vi "PQcopyOut.vi"(8 "error in (no error)":errorcluster, 9 "count":u32, 10 "query":string, 11 "conn":u32) -> (0 "database_status_message":T1, 1 "data":string[][](array[string]), 2 "column_names":string[](array[string]), 3 "conn_out":u32, 4 "error out":errorcluster)   [LabVIEW 2019, in "libpqutility.lvlib"]
doc: "Execute Command and get the result out with PQgetCopy \nonly usefull for COPY out Commands otherwise this VI does nothing then clearing the result\n!!!Make shure to set the 'Count' parameter on the amount of rows to expect in the result set!!!\n\nCOPY { tablename [ ( column [, ...] ) ] | ( query ) }\n TO { 'filename' | STDOUT }\n [ [ WITH ] \n [ BINARY ]\n [ HEADER ]\n [ OIDS ]\n [ DELIMITER [ AS ] 'delimiter' ]\n [ NULL [ AS ] 'null string' ]\n [ CSV [ HEADER ]\n [ QUOTE [ AS ] 'quote' ] \n [ ESCAPE [ AS ] 'escape' ]\n [ FORCE QUOTE column [, ...] ] \n \nSee PostgreSQL c-lib doku for further information."
uses:
  libpqutility.lvlib
  libpqlv/libpqlv.lvlib
panel:
  out "PQcmdTuples":string
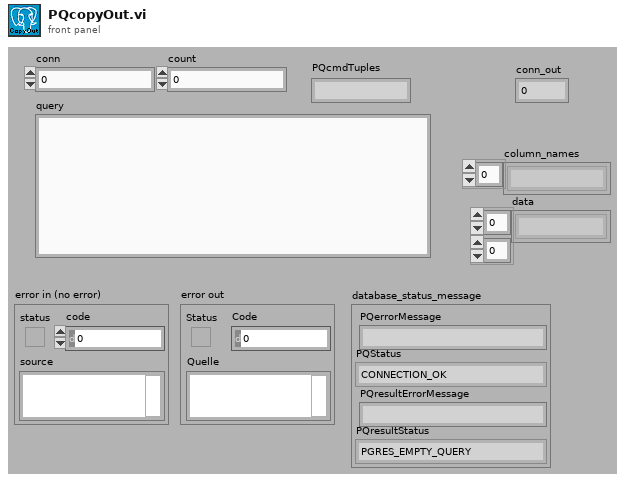
[diagram p1: front panel]
types:
  T1 = cluster{"PQerrorMessage":string, "PQStatus":enum16{"CONNECTION_OK", "CONNECTION_BAD", "CONNECTION_STARTED", "CONNECTION_MADE", "CONNECTION_AWAITING_RESPONSE", "CONNECTION_AUTH_OK", "CONNECTION_SETENV", "CONNECTION_SSL_STARTUP", "CONNECTION_NEEDED"}, "PQresultErrorMessage":string, "PQresultStatus":enum16{"PGRES_EMPTY_QUERY", "PGRES_COMMAND_OK", "PGRES_TUPLES_OK", "PGRES_COPY_OUT", "PGRES_COPY_IN", "PGRES_BAD_RESPONSE", "PGRES_NONFATAL_ERROR", "PGRES_FATAL_ERROR"}}
  T2 = enum32{"PGRES_EMPTY_QUERY", "PGRES_COMMAND_OK", "PGRES_TUPLES_OK", "PGRES_COPY_OUT", "PGRES_COPY_IN", "PGRES_BAD_RESPONSE", "PGRES_NONFATAL_ERROR", "PGRES_FATAL_ERROR"}
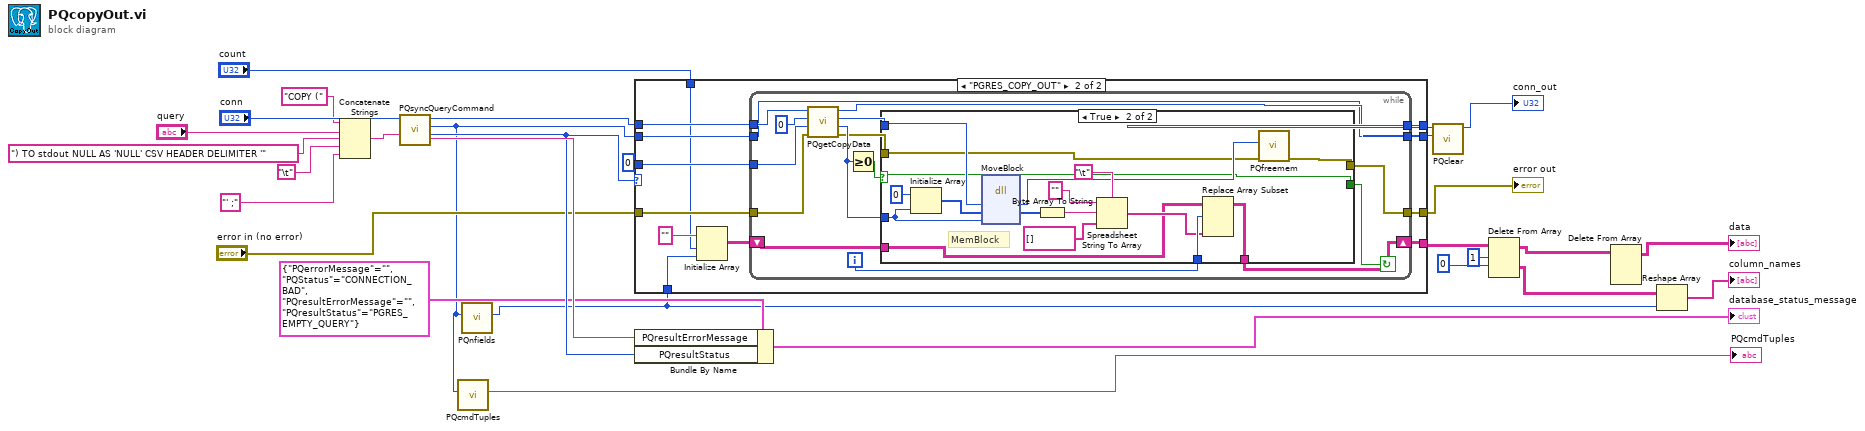
[diagram p0: block diagram]
diagram:
  n1 = Concatenate Strings("COPY (" ("String"), "query", ") TO stdout NULL AS 'NULL' CSV HEADER DELIMITER '" ("String"), "\t", "' ;" ("String")) -> (w11:string)
  n2 = call "PQsyncQueryCommand.vi"("query"=w11, "conn"="conn") -> ("PQresultStatus"=w24:T2, "PGresult"=w9:u32, "conn out"=w29:u32, "PQresultErrorMessage"=w25:string)  [unwired: 5 in, 1 out]
  n3 = call "PQcmdTuples.vi"("res"=w9) -> ("PQcmdTuples"=→"PQcmdTuples":string)  [unwired: 9 in, 1 out]
  n4 = call "PQnfields.vi"("res"=w9) -> ("res out"=w1:u32)  [unwired: 8 in, 2 out]
  n5 = case shown="\"PGRES_COPY_OUT\"" w24 {
    tunnel: w29 -> [w32 w44]
    tunnel: [w32 w43] -> w28
    tunnel: w9 -> [w31 w42]
    tunnel: [w31 w41] -> w27
    tunnel: [w30 w39] -> w26
    tunnel: 0 ("ptr") -> [_ w40]
    tunnel: "error in (no error)" -> [w30 w38]
    tunnel: [_ w37] -> w3
    tunnel: "count" -> [_ w34]
    tunnel: w1 -> [_ w33]
    frame Default {
    }
    frame "PGRES_COPY_OUT" {
      n6 = Initialize Array("" ("Format-String"), w34, w33) -> (w36:string[][])
      n7 = while {
        tunnel: w44 -> [w59]
        tunnel: [w58] -> w43
        tunnel: w42 -> [w57]
        tunnel: [w57] -> w41
        tunnel: w40 -> [w54]
        tunnel: [w49] -> w39
        tunnel: w38 -> [w48]
        shift-right: [w46] -> w37
        shift-left: w36 -> [w45]
        i -> [w47]
        stop <- w50 continue-if-true
        n8 = call "PQgetCopyData.vi"("error in (no error)"=w48, "async"=w54, "buffer"=u32 0 ("async"), "conn"=w59) -> ("error out"=w52:errorcluster, "PQgetCopyData"=w53:i32, "buffer_out"=w55:u32, "conn_out"=w58:u32)  [unwired: 4 in]
        n9 = Greater Or Equal To 0?(x=w53) -> (x >= 0?=w51:bool)
        n10 = case shown="True" w51 {
          selector: w51 -> [w61 w68]
          tunnel: w55 -> [_ w77]
          tunnel: w53 -> [_ w72]
          tunnel: w52 -> [w62 w70]
          tunnel: [w62 w69] -> w49
          tunnel: [w61 w68] -> w50
          tunnel: w47 -> [_ w66]
          tunnel: [w60 w64] -> w46
          tunnel: w45 -> [w60 w63]
          frame False {
          }
          frame True {
            # "MemBlock"
            n11 = Initialize Array(u8 0 ("ptr"), w72) -> (w78:u8[])
            n12 = dll-call lib="LabVIEW" fn="MoveBlock"("ps"=w77, "pd"=w78, "size_t"=w72) -> ("ps"=w71:u32, "pd"=w76:u8[])  [unwired: 5 in, 2 out]
            n13 = Byte Array To String(unsigned byte array=w76) -> (string=w74:string)
            n14 = Spreadsheet String To Array(delimiter (Tab)="\t" ("Trennzeichen (Tabulator)"), format string="" ("String"), spreadsheet string=w74, array type (2D Dbl)=string[] [] ("array")) -> (array=w65:string[])
            n15 = Replace Array Subset(array=w63, new element=w65, index (row)=w66) -> (w64:string[][])  [unwired: 1 in]
            n16 = call "PQfreemem.vi"("buffer"=w71, "error in (no error)"=w70) -> ("error out"=w69:errorcluster)  [unwired: 8 in]
          }
        }
      }
    }
  }
  "error out" <- w26
  n17 = Bundle By Name(cluster=T1 {"PQerrorMessage"="", "PQStatus"=enum."CONNECTION_BAD", "PQresultErrorMessage"="", "PQresultStatus"=enum."PGRES_EMPTY_QUERY"} ("Database Status Message 2"), "PQresultErrorMessage"=w25, "PQresultStatus"=w24) -> (→"database_status_message":T1)
  n18 = call "PQclear.vi"("res"=w27, "conn"=w28) -> ("conn_out"=→"conn_out":u32)  [unwired: 8 in, 1 out]
  n19 = Delete From Array(array=w3, length=1 ("Länge"), index (row)=0 ("Länge")) -> (deleted portion=w14:string[][], array with subset deleted=w5:string[][])  [unwired: 1 in]
  n20 = Delete From Array(array=w5) -> (array with subset deleted=→"data":string[][])  [unwired: 3 in, 1 out]
  n21 = Reshape Array(w14, w1) -> (→"column_names":string[])
